vi "ReadObjectLayout.vi"(7 "properties to ignore":variant, 8 "error in (no error)":errorcluster, 10 "GObj Refnum":refnum<vi>, 11 "Object Layout in":refnum<class "Pane Layout.lvclass">) -> (0 "error out":errorcluster, 3 "Object Layout out":refnum<class "Pane Layout.lvclass">)   [LabVIEW 2010, in "NI_SE_Front Panel Layout.lvlib" / "Pane Layout.lvclass"]
doc: "Read layout information from the GObj Refnum."
uses:
  Pane Layout.lvclass
  Object Layout/Object Layout.lvclass
  Pane Layout.lvclass/Pane Layout.ctl
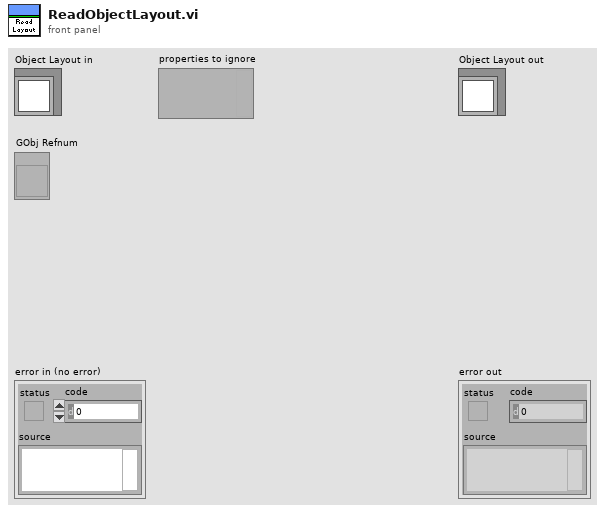
[diagram p1: front panel]
types:
  T1 = typedef "LVPointTypeDef.ctl" = cluster{"Horizontal":i16, "Vertical":i16}
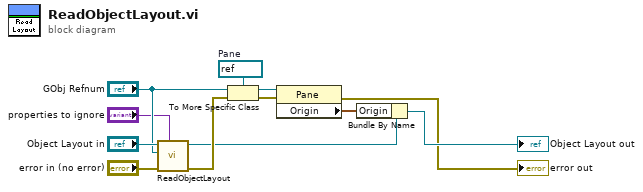
[diagram p0: block diagram]
diagram:
  w4 = refnum<vi> refnum  # Pane
  n1 = call-parent "ReadObjectLayout.vi"("properties to ignore"="properties to ignore", "error in (no error)"="error in (no error)", "GObj Refnum"="GObj Refnum", "Object Layout in"="Object Layout in") -> ("error out"=w10:errorcluster, "Object Layout out"=w9:refnum<class "Pane Layout.lvclass">)  [unwired: 6 in]
  n2 = To More Specific Class(target class=w4, reference="GObj Refnum", error in=w10) -> (specific class reference=w3:refnum<vi>, error out=w2:errorcluster)
  n3 = property class="Pane"(reference=w3, error in=w2) -> (error out=→"error out":errorcluster, "Origin"=w1:T1)  [unwired: 1 out]
  n4 = Bundle By Name(cluster=w9, "Origin"=w1) -> (→"Object Layout out":refnum<class "Pane Layout.lvclass">)
